vi "IFNoise-Analyze.vi"(0 "Runtime":T2, 9 "Params":T1={"Averages"=128, "Probe Mic Gain (dB)"=0.0, "Cal Mic Gain (dB)"=0.0, "Cal Mic Sens (dB V/SPL)"=0.0, "Attenuation (dB)"=20.0, "Sample size (s)"=128.0, "Input"=enum."Probe Mic"}, 11 "error in (no error)":errorcluster) -> (4 "Runtime out":T2, 8 "Mic signal":dbl[](array[numeric]), 15 "error out":errorcluster)   [LabVIEW 2015]
uses:
  Type Defs/IFNoise-Runtime.ctl
  Type Defs/IFNoise-Params.ctl
  <vilib>/Analysis/4window.llb/Modified Bartlett-Hanning Window (DBL).vi
  <vilib>/Analysis/5stat.llb/RMS (DBL).vi
  Utility VIs/Math VIs/FFT x(t) to dB,Degrees (1D).vi
  Utility VIs/Math VIs/dB to Linear (1D).vi
  <vilib>/Analysis/NI_AALPro.lvlib
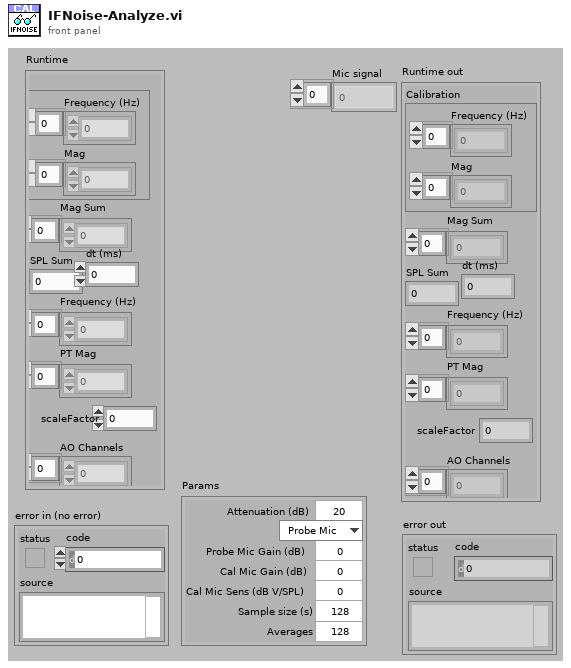
[diagram p1: front panel]
types:
  T1 = typedef "IFNoise-Params.ctl" = cluster{"Averages":i32, "Probe Mic Gain (dB)":dbl, "Cal Mic Gain (dB)":dbl, "Cal Mic Sens (dB V/SPL)":dbl, "Attenuation (dB)":dbl, "Sample size (s)":dbl, "Input":enum16{"Probe Mic", "Cal Mic", "Voltage Only"}}
  T2 = typedef "IFNoise-Runtime.ctl" = cluster{"Calibration":cluster{"Frequency (Hz)":dbl[], "Mag":dbl[]}, "Mag Sum":dbl[], "SPL Sum":dbl, "Frequency (Hz)":dbl[], "PT Mag":dbl[], "dt (ms)":dbl, "AO Channels":i32[], "scaleFactor":dbl}
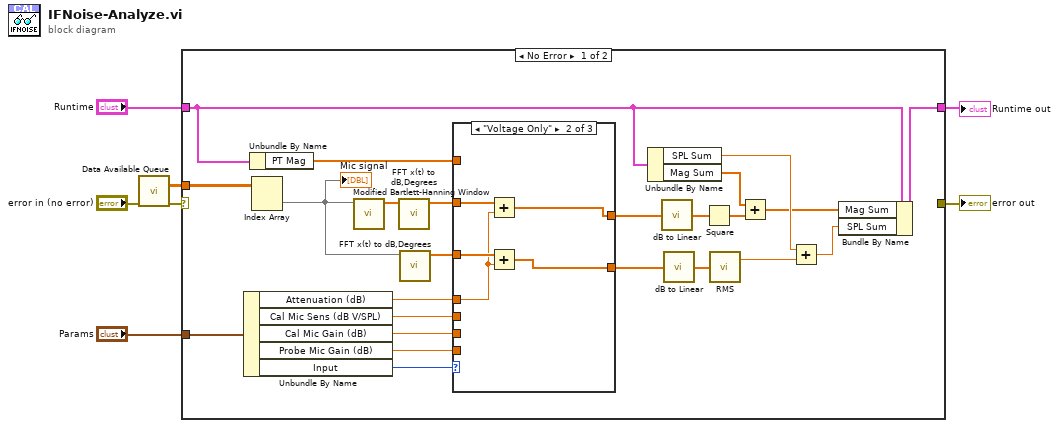
[diagram p0: block diagram]
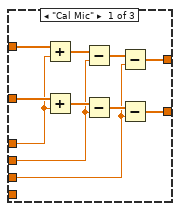
[diagram p2: hidden frame]
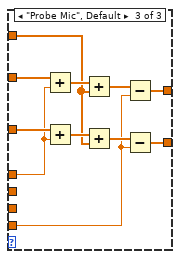
[diagram p3: hidden frame]
diagram:
  n1 = call "Data Available Queue.vi"("error in (no error)"="error in (no error)") -> ("Waveform Graph"=w2:dbl[][], "error out"=w4:errorcluster)  [unwired: 11 in, 2 out]
  n2 = case shown="No Error" w4 {
    selector: w4 -> [_ w60]
    tunnel: [_ w60] -> w7
    tunnel: "Runtime" -> [w13 w59]
    tunnel: "Params" -> [w28 _]
    tunnel: w2 -> [w14 _]
    tunnel: [w12 w59] -> w1
    frame No Error {
      n3 = Unbundle By Name(w28) -> ("Attenuation (dB)"=w21:dbl, "Cal Mic Sens (dB V/SPL)"=w23:dbl, "Cal Mic Gain (dB)"=w22:dbl, "Probe Mic Gain (dB)"=w20:dbl, "Input"=w27:enum16{"Probe Mic", "Cal Mic", "Voltage Only"})
      n4 = Unbundle By Name(w13) -> ("PT Mag"=w24:dbl[])
      n5 = Index Array(array=w14) -> (element=w9:dbl[])  [unwired: 2 in]
      "Mic signal" <- w9
      n6 = call-poly <vilib>:"Modified Bartlett-Hanning Window.vi"("X"=w9) -> ("Windowed X"=w8:dbl[])  [unwired: 9 in, 1 out]
      n7 = call-poly "FFT x(t) to dB,Degrees.vi"("X"=w8) -> ("+Freq. Mag of FFT (dB rms)"=w26:dbl[])  [unwired: 8 in, 2 out]
      n8 = call-poly "FFT x(t) to dB,Degrees.vi"("X"=w9) -> ("+Freq. Mag of FFT (dB rms)"=w25:dbl[])  [unwired: 8 in, 2 out]
      n9 = case shown="\"Voltage Only\"" w27 {
        tunnel: w26 -> [w37 w46 w53]
        tunnel: w25 -> [w42 w47 w58]
        tunnel: w24 -> [_ _ w48]
        tunnel: w23 -> [w35 _ _]
        tunnel: w22 -> [w34 _ _]
        tunnel: w21 -> [w36 w45 w52]
        tunnel: [w33 w44 w51] -> w19
        tunnel: [w32 w43 w50] -> w18
        tunnel: w20 -> [_ _ w49]
        frame "Cal Mic" {
          n10 = Add(x=w37, y=w36) -> (x+y=w39:dbl[])
          n11 = Add(x=w42, y=w36) -> (x+y=w41:dbl[])
          n12 = Subtract(x=w39, y=w35) -> (x-y=w38:dbl[])
          n13 = Subtract(x=w41, y=w35) -> (x-y=w40:dbl[])
          n14 = Subtract(x=w38, y=w34) -> (x-y=w33:dbl[])
          n15 = Subtract(x=w40, y=w34) -> (x-y=w32:dbl[])
        }
        frame "Voltage Only" {
          n16 = Add(x=w46, y=w45) -> (x+y=w44:dbl[])
          n17 = Add(x=w47, y=w45) -> (x+y=w43:dbl[])
        }
        frame "Probe Mic", Default {
          n18 = Add(x=w53, y=w52) -> (x+y=w55:dbl[])
          n19 = Add(x=w58, y=w52) -> (x+y=w57:dbl[])
          n20 = Add(x=w55, y=w48) -> (x+y=w54:dbl[])
          n21 = Add(x=w57, y=w48) -> (x+y=w56:dbl[])
          n22 = Subtract(x=w54, y=w49) -> (x-y=w51:dbl[])
          n23 = Subtract(x=w56, y=w49) -> (x-y=w50:dbl[])
        }
      }
      n24 = Unbundle By Name(w13) -> ("SPL Sum"=w15:dbl, "Mag Sum"=w29:dbl[])
      n25 = call-poly "dB to Linear.vi"("dB"=w19) -> ("linear"=w31:dbl[])
      n26 = call-poly "dB to Linear.vi"("dB"=w18) -> ("linear"=w17:dbl[])
      n27 = Square(x=w31) -> (x^2=w30:dbl[])
      n28 = call-poly <vilib>:"RMS.vi"("X"=w17) -> ("rms value"=w16:dbl)  [unwired: 1 out]
      n29 = Add(x=w29, y=w30) -> (x+y=w11:dbl[])
      n30 = Add(x=w15, y=w16) -> (x+y=w10:dbl)
      n31 = Bundle By Name(cluster=w13, "Mag Sum"=w11, "SPL Sum"=w10) -> (w12:T2)
    }
    frame Error {
    }
  }
  "error out" <- w7
  "Runtime out" <- w1
